vi "B value From itx.vi"(11 "file (use dialog)":path) -> (3 "Numeric":dbl)   [LabVIEW 2016]
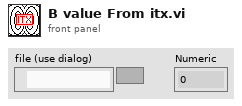
[diagram p1: front panel]
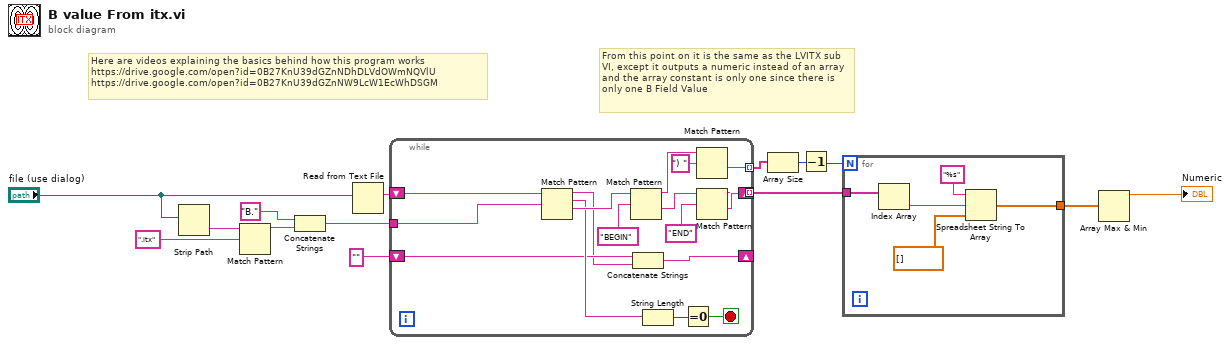
[diagram p0: block diagram]
diagram:
  # "Here are videos explaining the basics behind how this program works\nhttps://drive.google.com/open?id=0B27KnU39dGZnNDhDLVdOWmNQVlU\nhttps://drive.google.com/open?id=0B27KnU39dGZnNW9LcW1EcWhDSGM"
  # "From this point on it is the same as the LVITX sub VI, except it outputs a numeric instead of an array and the array constant is only one since there is only one B Field Value"
  n1 = Strip Path(path="file (use dialog)") -> (name=w3:string)  [unwired: 1 out]
  n2 = Match Pattern(string=w3, regular expression=".itx") -> (before substring=w2:string)  [unwired: 1 in, 3 out]
  n3 = Concatenate Strings("B." ("string"), w2) -> (w1:string)
  n4 = Read from Text File(file (use dialog)="file (use dialog)") -> (text=w12:string)  [unwired: 2 in, 4 out]
  n5 = while {
    tunnel: [w16] -> w10 mode=indexing
    shift-right: [w29] -> _
    shift-left: w12 -> [w18]
    tunnel: [w25] -> w9 mode=indexing
    shift-right: [w21] -> _
    shift-left: "" ("regular expression") -> [w20]
    tunnel: w1 -> [w15]
    stop <- w26 stop-if-true
    n6 = Match Pattern(string=w18, regular expression=w15) -> (before substring=w19:string, match substring=w28:string, after substring=w31:string)  [unwired: 2 out]
    n7 = Match Pattern(string=w31, regular expression="BEGIN" ("regular expression 2")) -> (before substring=w17:string, after substring=w30:string)  [unwired: 3 out]
    n8 = Concatenate Strings(w20, w19) -> (w21:string)
    n9 = String Length(string=w28) -> (length=w27:i32)
    n10 = Equal To 0?(x=w27) -> (x = 0?=w26:bool)
    n11 = Match Pattern(string=w17, regular expression=") ") -> (after substring=w25:string)  [unwired: 4 out]
    n12 = Match Pattern(string=w30, regular expression="END" ("regular expression 3")) -> (before substring=w16:string, after substring=w29:string)  [unwired: 3 out]
  }
  n13 = Array Size(array=w9) -> (size(s)=w8:i32)
  n14 = Decrement(x=w8) -> (x-1=w7:i32)
  n15 = for {
    N: w7 -> [_]
    tunnel: w10 -> [w36]
    tunnel: [w32] -> w13
    n16 = Index Array(array=w36) -> (element=w35:string)  [unwired: 1 in]
    n17 = Spreadsheet String To Array(format string="%s", spreadsheet string=w35, array type (2D Dbl)=dbl[] []) -> (array=w32:dbl[])  [unwired: 1 out]
  }
  n18 = Array Max & Min(array=w13) -> (max value=→"Numeric":dbl)  [unwired: 3 out]
